vi "Aim via Speed.vi"(2 "Angle(degrees)":dbl=45.0, 3 "Vision Distance(in)":dbl=120.0) -> (0 "error out":errorcluster, 1 "Initial Speed(in/s)":dbl)   [LabVIEW 2015]
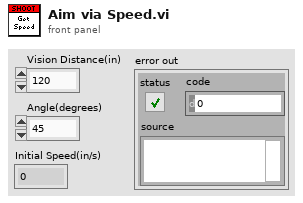
[diagram p1: front panel]
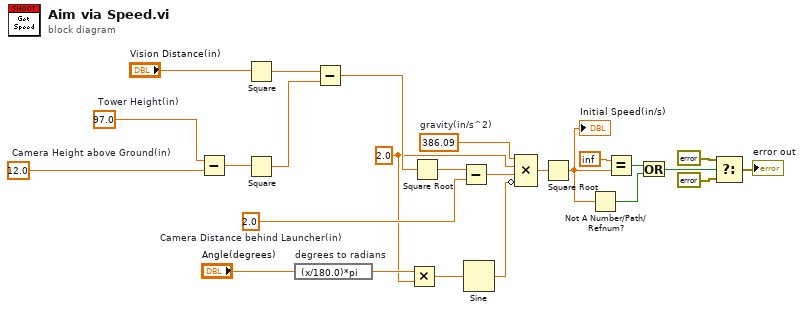
[diagram p0: block diagram]
diagram:
  w10 = 386.09  # gravity(in/s^2)
  w9 = 2.0 ("y")
  w24 = 2.0  # Camera Distance behind Launcher(in)
  w22 = 12.0  # Camera Height above Ground(in)
  w23 = 97.0  # Tower Height(in)
  n1 = Subtract(x=w23, y=w22) -> (x-y=w25:dbl)
  n2 = Square(x="Vision Distance(in)") -> (x^2=w18:dbl)
  n3 = Square(x=w25) -> (x^2=w19:dbl)
  n4 = expression code="(x/180.0)*pi" "degrees to radians"("Angle(degrees)") -> (w13:dbl)
  n5 = Subtract(x=w18, y=w19) -> (x-y=w20:dbl)
  n6 = Multiply(x=w13, y=w9) -> (x*y=w12:dbl)
  n7 = Square Root(x=w20) -> (sqrt(x)=w17:dbl)
  n8 = Subtract(x=w17, y=w24) -> (x-y=w7:dbl)
  n9 = Sine(x=w12) -> (sin(x)=w11:dbl)
  n10 = Compound Arithmetic op=MULTIPLY(w10, w9, w7, invert w11) -> (w8:dbl)
  n11 = Square Root(x=w8) -> (sqrt(x)=w5:dbl)
  "Initial Speed(in/s)" <- w5
  n12 = Not A Number/Path/Refnum?(number/path/refnum=w5) -> (NaN/Path/Refnum?=w3:bool)
  n13 = Equal?(x=inf, y=w5) -> (x = y?=w4:bool)
  n14 = Or(x=w4, y=w3) -> (x .or. y?=w2:bool)
  n15 = Select(t=errorcluster {"status"=TRUE, "code"=9002, "source"="Invalid launch angle!"} ("error constant"), s=w2, f=errorcluster {"status"=FALSE, "code"=0, "source"=""}) -> (s? t:f=→"error out":errorcluster)
